vi "FPGA Globals.vi"() -> ()   [LabVIEW 2014]
panel:
  out "Error":bool
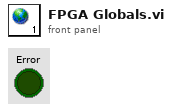
[diagram p1: front panel]
diagram:
